vi "score generator.vi"(1 "Numeric 2":dbl=20.0, 2 "Numeric":dbl=80.0) -> (0 "Numeric 3":dbl)   [LabVIEW 2014]
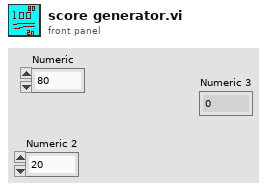
[diagram p1: front panel]
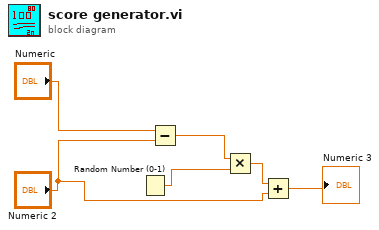
[diagram p0: block diagram]
diagram:
  n1 = Random Number (0-1)() -> (number: 0 to 1=w5:dbl)
  n2 = Subtract(x="Numeric", y="Numeric 2") -> (x-y=w4:dbl)
  n3 = Multiply(x=w4, y=w5) -> (x*y=w3:dbl)
  n4 = Add(x=w3, y="Numeric 2") -> (x+y=→"Numeric 3":dbl)
